vi "XNET Create Timing Source.vi"   [LabVIEW 2018]
doc: "Creates a timing source for a Timed Loop on LabVIEW Real-Time.\n\nThe instances of this polymorphic VI specify the type of timing source."
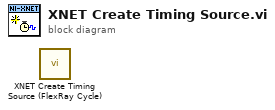
[diagram p0: block diagram]
diagram:
  n1 = call "XNET Create Timing Source (FlexRay Cycle).vi"() -> ()  [unwired: 13 in, 3 out]
